vi "FTW-STR-Encode-Hex.vi"(0 "Input":string, 1 "Direction":enum16{"Encode", "Decode"}(ring)) -> (2 "Output":string)   [LabVIEW 2013]
panel:
  # "Inputs"
  # "Outputs"
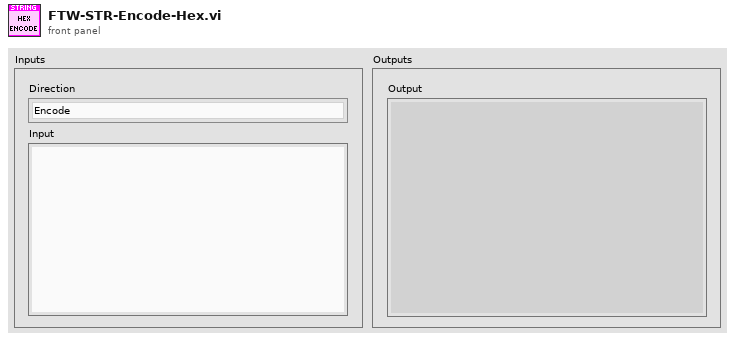
[diagram p1: front panel]
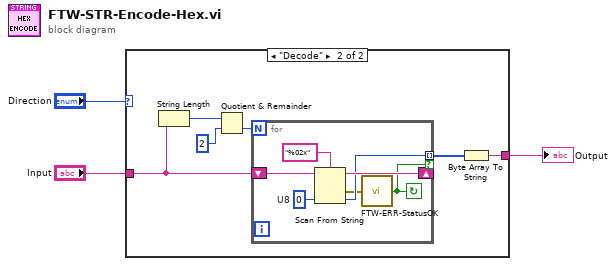
[diagram p0: block diagram]
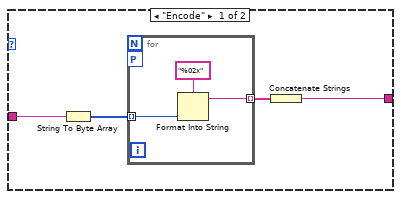
[diagram p2: hidden frame]
diagram:
  n1 = case shown="\"Decode\"" "Direction" {
    tunnel: [w5 w15] -> w1
    tunnel: "Input" -> [w6 w14]
    frame "Encode" {
      n2 = String To Byte Array(string=w6) -> (unsigned byte array=w7:u8[])
      n3 = for {
        tunnel: [w9] -> w4 mode=indexing
        tunnel: w7 -> [w8] mode=indexing
        workers-P: _ -> [_]
        n4 = Format Into String(format string="%02x", w8) -> (resulting string=w9:string)  [unwired: 2 in, 1 out]
      }
      n5 = Concatenate Strings(w4) -> (w5:string)
    }
    frame "Decode" {
      n6 = String Length(string=w14) -> (length=w13:i32)
      n7 = Quotient & Remainder(x=w13, y=2) -> (floor(x/y)=w11:i32)  [unwired: 1 out]
      n8 = for {
        N: w11 -> [_]
        shift-right: [w21] -> _
        shift-left: w14 -> [w22]
        tunnel: [w19] -> w16 mode=indexing if=w17
        stop <- w17 continue-if-true
        w20 = u8 0  # U8
        n9 = Scan From String(format string="%02x", input string=w22, default 1=w20) -> (remaining string=w21:string, error out=w18:errorcluster, output 1=w19:u8)  [unwired: 2 in, 1 out]
        n10 = call "FTW-ERR-StatusOK.vi"("error to check"=w18) -> ("Status OK?"=w17:bool)
      }
      n11 = Byte Array To String(unsigned byte array=w16) -> (string=w15:string)
    }
  }
  "Output" <- w1
